vi "Get Scaling Parameters (Linear).vi"(0 "session in":refnum<k21>, 5 "physical channel":refnum<k21>="$DefaultPhysChans", 11 "error in (no error)":errorcluster) -> (4 "session out":refnum<k21>, 6 "physical channel out":refnum<k21>, 8 "slope":dbl, 10 "intercept":dbl, 15 "error out":errorcluster)   [LabVIEW 2020, in "SLSC.lvlib"]
doc: "Gets scaling parameters from a linear scale that uses the equation y = mx + b, where x is a pre-scaled value and y is a scaled value."
uses:
  <vilib>/SLSC/SLSC.lvlib
  nislsclvapi.dll
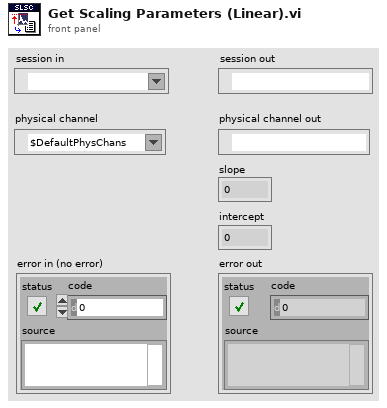
[diagram p1: front panel]
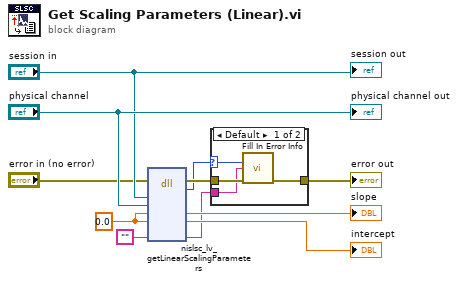
[diagram p0: block diagram]
diagram:
  w1 = 0.0 ("slope")
  n1 = dll-call lib="nislsclvapi.*" fn="nislsc_lv_getLinearScalingParameters"(error in="error in (no error)", "session"="session in", "physical channel"="physical channel", "slope"=w1, "intercept"=w1, "extendedErrorInfo"="") -> (error out=w4:errorcluster, "return type"=w2:i32, "slope"=→"slope":dbl, "intercept"=→"intercept":dbl, "extendedErrorInfo"=w3:string)  [unwired: 6 in, 1 out]
  n2 = case shown="Default" w2 {
    selector: w2 -> [w12 _]
    tunnel: w3 -> [w13 _]
    tunnel: w4 -> [w15 w16]
    tunnel: [w14 w16] -> w5
    frame Default {
      n3 = call <vilib>:"Fill In Error Info.vi"("status code"=w12, "extended error info"=w13, "error in"=w15) -> ("error out"=w14:errorcluster)  [unwired: 12 in]
    }
    frame 0 {
    }
  }
  "error out" <- w5
  "session out" <- "session in"
  "physical channel out" <- "physical channel"
